vi "HV_VSet_Single.vi"(8 "Voltage":string, 11 "Channel":string) -> (3 "standard output":string)   [LabVIEW 2019]
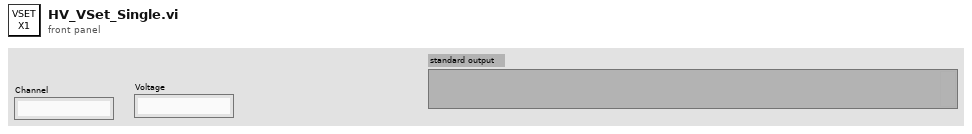
[diagram p1: front panel]
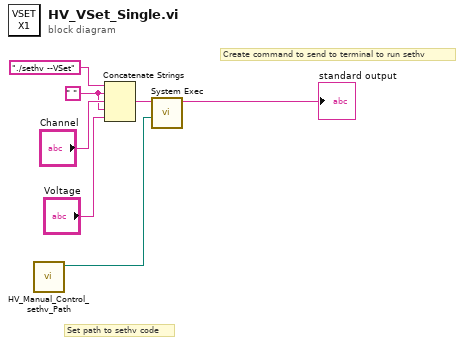
[diagram p0: block diagram]
diagram:
  w4 = " " ("string")
  # "Create command to send to terminal to run sethv"
  # "Set path to sethv code"
  n1 = call "HV_Manual_Control_sethv_Path.vi"() -> ("sethv filepath"=w1:path)  [unwired: 11 in]
  n2 = Concatenate Strings("./sethv --VSet" ("string"), w4, "Channel", w4, "Voltage") -> (w7:string)
  n3 = call <vilib>:"System Exec.vi"("working directory"=w1, "command line"=w7) -> ("standard output"=→"standard output":string)  [unwired: 6 in, 3 out]
